vi "XIPIN_Partial_Reconfiguration_Controller_1_0.vi"   [LabVIEW 2017]
doc: "The Partial Reconfiguration Controller provides a hardware block to manage the loading and removal of Reconfigurable Modules via the ICAP port\n------------------------------------\n<b>Need License</b> : No"
uses:
  <vilib>/rvi/XilinxIP/XIPIN_XNode/niFpgaXIPIN.xnode
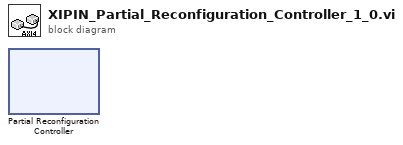
[diagram p0: block diagram]
diagram:
  n1 = xnode ("Partial Reconfiguration Controller")() -> ()
